vi "质控单元3流程.vi"   [LabVIEW 2016]
types:
  T1 = enum16{"步骤1", "步骤2", "步骤3", "步骤4", "步骤5", "步骤6", "步骤7", "步骤8", "步骤9", "步骤10"}
  T2 = enum32{"Bad", "Idle", "Run top level", "Running"}
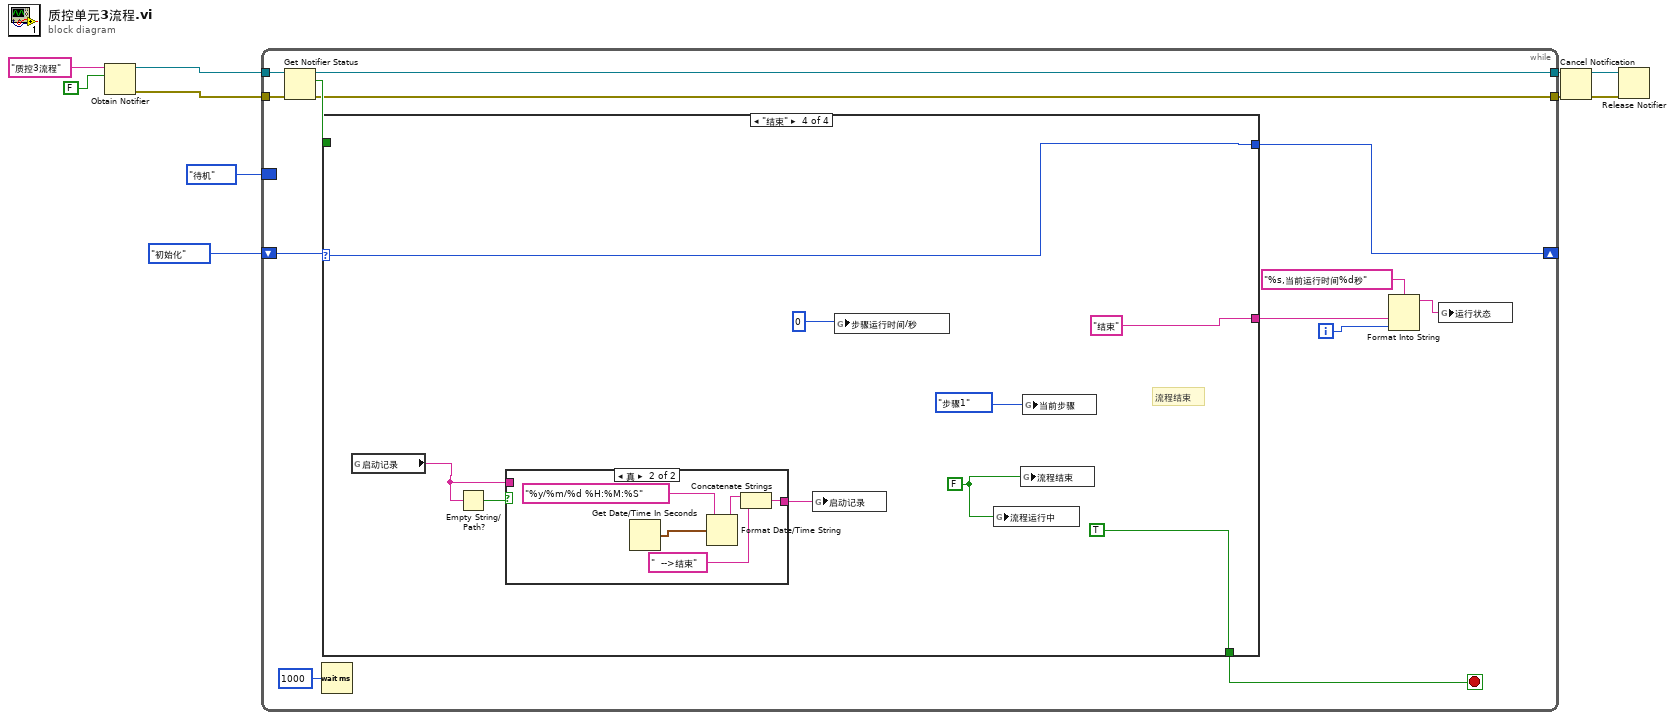
[diagram p0: block diagram]
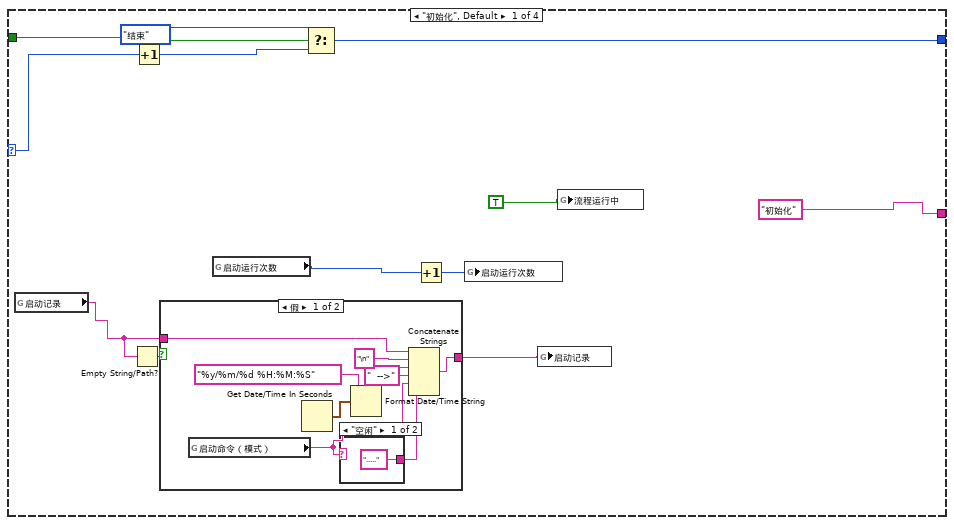
[diagram p2: hidden frame]
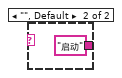
[diagram p3: hidden frame]
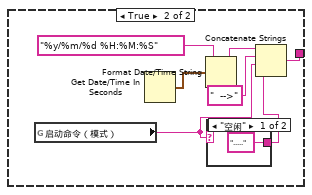
[diagram p4: hidden frame]
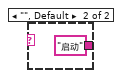
[diagram p5: hidden frame]
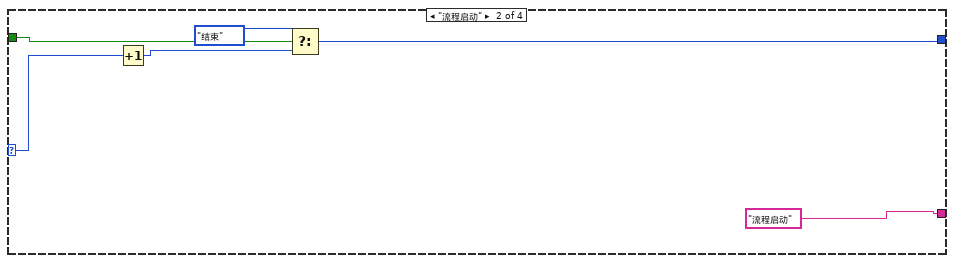
[diagram p6: hidden frame]
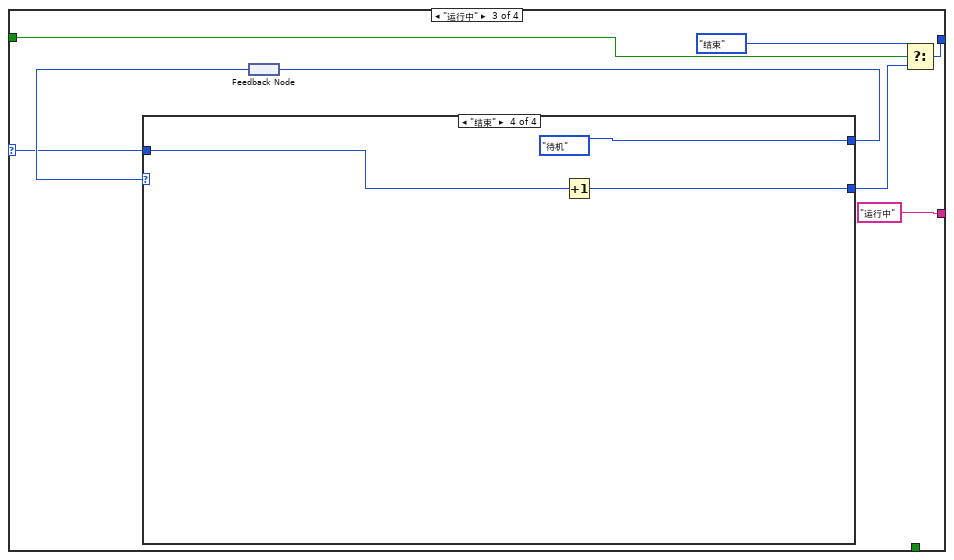
[diagram p7: hidden frame]
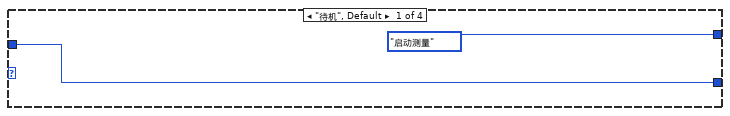
[diagram p8: hidden frame]
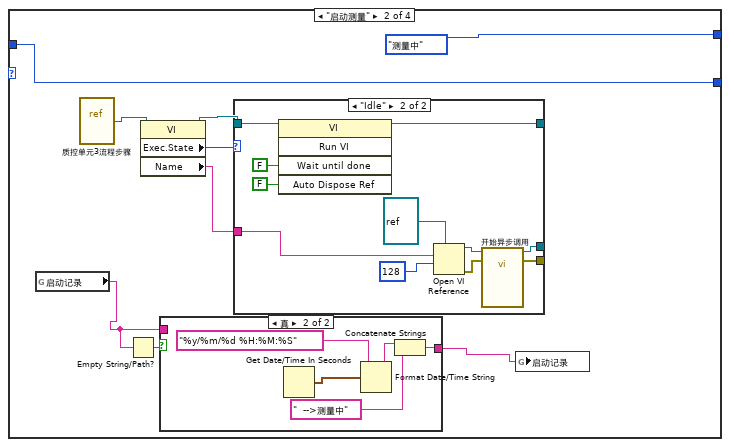
[diagram p9: hidden frame]
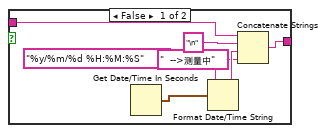
[diagram p10: hidden frame]
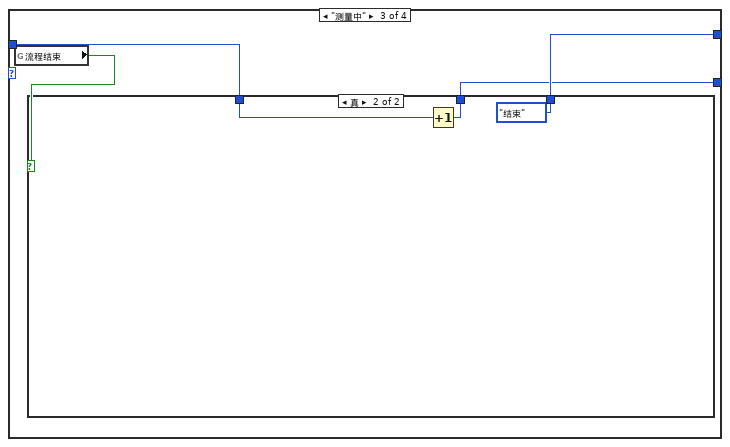
[diagram p12: hidden frame]
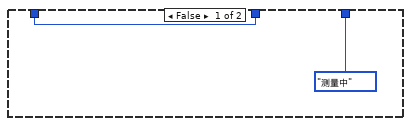
[diagram p13: hidden frame]
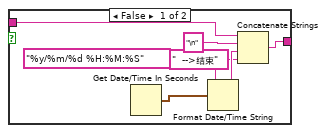
[diagram p14: hidden frame]
diagram:
  n1 = Obtain Notifier(name (unnamed)="质控3流程" ("名称（未命名）"), notification data type=FALSE) -> (notifier out=w7:refnum<notifier>, error out=w6:errorcluster)  [unwired: 2 in, 1 out]
  n2 = while {
    shift-right: [w20] -> _
    shift-left: enum16{"初始化", "流程启动", "运行中", "结束"}."初始化" ("枚举") -> [w23]
    tunnel: w7 -> [w15]
    tunnel: w6 -> [w14]
    tunnel: [w13] -> w5
    tunnel: [w12] -> w4
    border: enum16{"待机", "启动测量", "测量中", "结束"}."待机" -> [_]
    i -> [w18]
    stop <- w16 stop-if-true
    n3 = Get Notifier Status(notifier=w15, error in (no error)=w14) -> (notifier out=w13:refnum<notifier>, current notification=w21:bool, error out=w12:errorcluster)  [unwired: 2 out]
    n4 = Wait (ms)(milliseconds to wait=u32 1000 ("等待时间（毫秒）")) -> ()  [unwired: 1 out]
    n5 = case shown="\"结束\"" w23 {
      selector: w23 -> [w33 w58 w64 w123]
      tunnel: [_ _ _ TRUE ("x")] -> w16
      tunnel: w21 -> [w35 w59 w68 _]
      tunnel: [w31 w57 w63 w123] -> w20
      tunnel: ["初始化" ("输入 1") "流程启动" ("输入 1") "运行中" ("输入 1") "结束" ("输入 1")] -> w17
      frame "初始化", Default {
        n6 = global read "质控单元3全局.vi" "启动记录"() -> (w27:string)
        n7 = Empty String/Path?(string/path=w27) -> (empty?=w29:bool)
        n8 = Increment(x=w33) -> (x+1=w32:enum16{"初始化", "流程启动", "运行中", "结束"})
        n9 = case shown="假" w29 {
          tunnel: w27 -> [w44 _]
          tunnel: [w39 w50] -> w28
          frame False {
            n10 = global read "质控单元3全局.vi" "启动命令（模式）"() -> (w36:string)
            n11 = Get Date/Time In Seconds() -> (seconds since 1Jan1904=w42:timestamp)
            n12 = case shown="\"空闲\"" w36 {
              tunnel: ["....." ("字符串") "启动" ("字符串")] -> w37
              frame "空闲" {
              }
              frame "", Default {
              }
            }
            n13 = Format Date/Time String(time format string (%c)="%y/%m/%d %H:%M:%S" ("时间格式字符串(%c)"), seconds (now)=w42) -> (date/time string=w40:string)  [unwired: 1 in]
            n14 = Concatenate Strings(w44, "\n" ("字符串"), w40, "  -->" ("字符串"), w36, w37) -> (w39:string)
          }
          frame True {
            n15 = global read "质控单元3全局.vi" "启动命令（模式）"() -> (w47:string)
            n16 = Get Date/Time In Seconds() -> (seconds since 1Jan1904=w53:timestamp)
            n17 = Format Date/Time String(time format string (%c)="%y/%m/%d %H:%M:%S" ("时间格式字符串(%c)"), seconds (now)=w53) -> (date/time string=w51:string)  [unwired: 1 in]
            n18 = case shown="\"空闲\"" w47 {
              tunnel: ["....." ("字符串") "启动" ("字符串")] -> w48
              frame "空闲" {
              }
              frame "", Default {
              }
            }
            n19 = Concatenate Strings(w51, "  -->" ("字符串"), w47, w48) -> (w50:string)
          }
        }
        n20 = global read "质控单元3全局.vi" "启动运行次数"() -> (w26:i32)
        n21 = Select(t=enum16{"初始化", "流程启动", "运行中", "结束"}."结束" ("枚举"), s=w35, f=w32) -> (s? t:f=w31:enum16{"初始化", "流程启动", "运行中", "结束"})
        n22 = Increment(x=w26) -> (x+1=w25:i32)
        n23 = global write "质控单元3全局.vi" "启动运行次数"(w25) -> ()
        n24 = global write "质控单元3全局.vi" "启动记录"(w28) -> ()
        n25 = global write "质控单元3全局.vi" "流程运行中"(TRUE ("流程运行中")) -> ()
      }
      frame "流程启动" {
        n26 = Increment(x=w58) -> (x+1=w60:enum16{"初始化", "流程启动", "运行中", "结束"})
        n27 = Select(t=enum16{"初始化", "流程启动", "运行中", "结束"}."结束" ("枚举"), s=w59, f=w60) -> (s? t:f=w57:enum16{"初始化", "流程启动", "运行中", "结束"})
      }
      frame "运行中" {
        n28 = feedback #1() -> (w67:enum16{"待机", "启动测量", "测量中", "结束"})
        n29 = case shown="\"结束\"" w67 {
          tunnel: [enum16{"待机", "启动测量", "测量中", "结束"}."启动测量" enum16{"待机", "启动测量", "测量中", "结束"}."测量中" w108 enum16{"待机", "启动测量", "测量中", "结束"}."待机"] -> w66
          tunnel: [w70 w79 w106 w115] -> w65
          tunnel: w64 -> [w70 w79 w107 w114]
          frame "待机", Default {
          }
          frame "启动测量" {
            n30 = global read "质控单元3全局.vi" "启动记录"() -> (w73:string)
            n31 = vi-ref "质控单元3流程步骤.vi"() -> (w75:refnum<vi>)
            n32 = Empty String/Path?(string/path=w73) -> (empty?=w74:bool)
            n33 = property class="VI"(reference=w75) -> (reference out=w76:refnum<vi>, "Exec.State"=w77:T2, "Name"=w78:string)  [unwired: 1 in, 1 out]
            n34 = case shown="真" w74 {
              tunnel: w73 -> [w87 _]
              tunnel: [w81 w88] -> w72
              frame False {
                n35 = Get Date/Time In Seconds() -> (seconds since 1Jan1904=w85:timestamp)
                n36 = Format Date/Time String(time format string (%c)="%y/%m/%d %H:%M:%S" ("时间格式字符串(%c)"), seconds (now)=w85) -> (date/time string=w83:string)  [unwired: 1 in]
                n37 = Concatenate Strings(w87, "\n" ("字符串"), w83, "  -->测量中" ("字符串")) -> (w81:string)
              }
              frame True {
                n38 = Get Date/Time In Seconds() -> (seconds since 1Jan1904=w92:timestamp)
                n39 = Format Date/Time String(time format string (%c)="%y/%m/%d %H:%M:%S" ("时间格式字符串(%c)"), seconds (now)=w92) -> (date/time string=w90:string)  [unwired: 1 in]
                n40 = Concatenate Strings(w90, "  -->测量中" ("字符串")) -> (w88:string)
              }
            }
            n41 = case shown="\"Idle\"" w77 {
              tunnel: w76 -> [w93 w101]
              tunnel: [w93 w102] -> _
              tunnel: w78 -> [_ w100]
              tunnel: [_ w95] -> _
              tunnel: [_ w94] -> _
              frame "Bad", Default {
              }
              frame "Idle" {
                n42 = invoke class="VI" method="Run VI"(reference=w101, "Wait until done"=FALSE ("结束前等待"), "Auto Dispose Ref"=FALSE ("自动销毁引用")) -> (reference out=w102:refnum<vi>)  [unwired: 2 in, 4 out]
                n43 = Open VI Reference(type specifier VI Refnum (for type only)=refnum<vi> refnum ("类型说明符VI引用句柄（仅用于类型）"), vi path=w100, options=128 ("选项")) -> (vi reference=w96:refnum<vi>, error out=w98:errorcluster)  [unwired: 3 in]
                n44 = call-by-ref "开始异步调用"(reference=w96, error in=w98) -> (reference out=w95:refnum<vi>, error out=w94:errorcluster)  [unwired: 12 in]
              }
            }
            n45 = global write "质控单元3全局.vi" "启动记录"(w72) -> ()
          }
          frame "测量中" {
            n46 = global read "质控单元3全局.vi" "流程结束"() -> (w105:bool)
            n47 = case shown="真" w105 {
              tunnel: [enum16{"待机", "启动测量", "测量中", "结束"}."测量中" enum16{"待机", "启动测量", "测量中", "结束"}."结束"] -> w108
              tunnel: w107 -> [w109 w112]
              tunnel: [w109 w111] -> w106
              frame False {
              }
              frame True {
                n48 = Increment(x=w112) -> (x+1=w111:enum16{"初始化", "流程启动", "运行中", "结束"})
              }
            }
          }
          frame "结束" {
            n49 = Increment(x=w114) -> (x+1=w115:enum16{"初始化", "流程启动", "运行中", "结束"})
          }
        }
        n50 = feedback-in #1(w66) -> ()
        n51 = Select(t=enum16{"初始化", "流程启动", "运行中", "结束"}."结束" ("枚举"), s=w68, f=w65) -> (s? t:f=w63:enum16{"初始化", "流程启动", "运行中", "结束"})
      }
      frame "结束" {
        w118 = FALSE ("流程结束")
        # "流程结束"
        n52 = global read "质控单元3全局.vi" "启动记录"() -> (w120:string)
        n53 = Empty String/Path?(string/path=w120) -> (empty?=w122:bool)
        n54 = case shown="真" w122 {
          tunnel: w120 -> [w132 _]
          tunnel: [w126 w133] -> w121
          frame False {
            n55 = Get Date/Time In Seconds() -> (seconds since 1Jan1904=w130:timestamp)
            n56 = Format Date/Time String(time format string (%c)="%y/%m/%d %H:%M:%S" ("时间格式字符串(%c)"), seconds (now)=w130) -> (date/time string=w128:string)  [unwired: 1 in]
            n57 = Concatenate Strings(w132, "\n" ("字符串"), w128, "  -->结束" ("字符串")) -> (w126:string)
          }
          frame True {
            n58 = Get Date/Time In Seconds() -> (seconds since 1Jan1904=w137:timestamp)
            n59 = Format Date/Time String(time format string (%c)="%y/%m/%d %H:%M:%S" ("时间格式字符串(%c)"), seconds (now)=w137) -> (date/time string=w135:string)  [unwired: 1 in]
            n60 = Concatenate Strings(w135, "  -->结束" ("字符串")) -> (w133:string)
          }
        }
        n61 = global write "质控单元3全局.vi" "启动记录"(w121) -> ()
        n62 = global write "质控单元3全局.vi" "步骤运行时间/秒"(0 ("运行时间/秒")) -> ()
        n63 = global write "质控单元3全局.vi" "流程运行中"(w118) -> ()
        n64 = global write "质控单元3全局.vi" "流程结束"(w118) -> ()
        n65 = global write "质控单元3全局.vi" "当前步骤"(T1."步骤1" ("当前步骤 2")) -> ()
      }
    }
    n66 = Format Into String(format string="%s,当前运行时间%d秒" ("格式字符串"), w17, w18) -> (resulting string=w11:string)  [unwired: 2 in, 1 out]
    n67 = global write "质控单元3全局.vi" "运行状态"(w11) -> ()
  }
  n68 = Cancel Notification(0:w5, 3:w4) -> (8:w3:refnum<notifier>, 11:w2:errorcluster)  [unwired: 1 out]
  n69 = Release Notifier(notifier=w3, error in (no error)=w2) -> ()  [unwired: 1 in, 3 out]
